vi "Degree_To_Bit_Conversion_Stream_Data_Generation.vi"(9 "Reset To Zero?":bool, 10 "Degree":dbl[](array[numeric])) -> (2 "Commands":T1(array[cluster]))   [LabVIEW 2015]
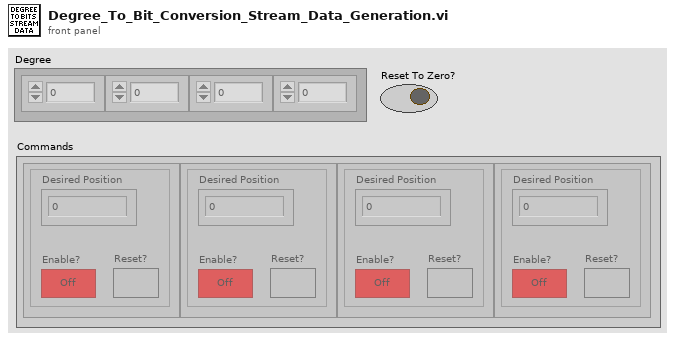
[diagram p1: front panel]
types:
  T1 = cluster{"Desired Position":u16, "Enable?":bool, "Reset?":bool}[]
  T2 = cluster{"Desired Position":u16, "Enable?":bool, "Reset?":bool}
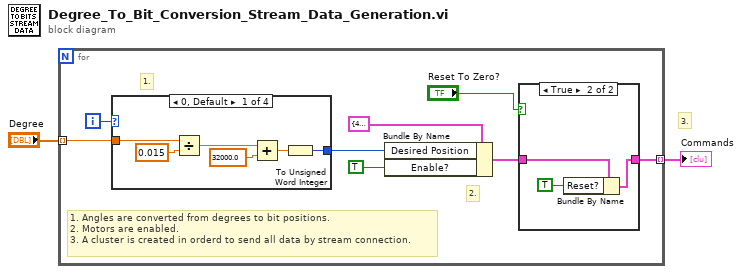
[diagram p0: block diagram]
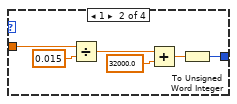
[diagram p3: hidden frame]
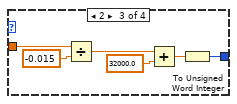
[diagram p4: hidden frame]
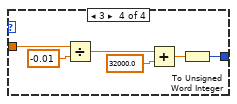
[diagram p5: hidden frame]
diagram:
  # "3."
  n1 = for {
    tunnel: "Degree" -> [w9] mode=indexing
    tunnel: [w4] -> w1 mode=indexing
    i -> [w10]
    # "2."
    # "1."
    # "1. Angles are converted from degrees to bit positions.\n2. Motors are enabled.\n3. A cluster is created in orderd to send all data by stream connection."
    n2 = case shown="0, Default" w10 {
      tunnel: w9 -> [w20 w22 w28 w34]
      tunnel: [w15 w21 w27 w33] -> w6
      frame 0, Default {
        n3 = Divide(x=w20, y=0.015) -> (x/y=w18:dbl)
        n4 = Add(x=w18, y=32000.0) -> (x+y=w16:dbl)
        n5 = To Unsigned Word Integer(number=w16) -> (unsigned 16bit integer=w15:u16)
      }
      frame 1 {
        n6 = Divide(x=w22, y=0.015) -> (x/y=w24:dbl)
        n7 = Add(x=w24, y=32000.0) -> (x+y=w26:dbl)
        n8 = To Unsigned Word Integer(number=w26) -> (unsigned 16bit integer=w21:u16)
      }
      frame 2 {
        n9 = Divide(x=w28, y=-0.015) -> (x/y=w30:dbl)
        n10 = Add(x=w30, y=32000.0) -> (x+y=w32:dbl)
        n11 = To Unsigned Word Integer(number=w32) -> (unsigned 16bit integer=w27:u16)
      }
      frame 3 {
        n12 = Divide(x=w34, y=-0.01) -> (x/y=w36:dbl)
        n13 = Add(x=w36, y=32000.0) -> (x+y=w38:dbl)
        n14 = To Unsigned Word Integer(number=w38) -> (unsigned 16bit integer=w33:u16)
      }
    }
    n15 = Bundle By Name(cluster=T2 {"Desired Position"=40000, "Enable?"=TRUE, "Reset?"=FALSE} ("Cluster"), "Desired Position"=w6, "Enable?"=TRUE) -> (w5:T2)
    n16 = case shown="True" "Reset To Zero?" {
      tunnel: w5 -> [w11 w14]
      tunnel: [w11 w12] -> w4
      frame False {
      }
      frame True {
        n17 = Bundle By Name(cluster=w14, "Reset?"=TRUE) -> (w12:T2)
      }
    }
  }
  "Commands" <- w1
